vi "[Alternate Method] Extract Data from N-Channel Array (1D Waveform).vi"() -> ()   [LabVIEW 2019]
uses:
  <vilib>/DAQmx/read.llb/DAQmx Read (Analog 1D Wfm NChan NSamp).vi
  <vilib>/DAQmx/create/channels.llb/DAQmx Create Channel (AI-Voltage-Basic).vi
  <vilib>/DAQmx/configure/timing.llb/DAQmx Timing (Sample Clock).vi
  <vilib>/DAQmx/miscellaneous.llb/DAQmx Fill In Error Info.vi
  <resource>/objmgr/daqmx.rc
panel:
  out "Actual Sample Rate (Hz)":dbl
  in  "Desired Sample Rate (Hz)":dbl=2560.0
  in  "Number of Samples":i32=256
  in  "Stop":bool
  out "All Channels":waveform(dbl)[](graph)
  out "Indexed Channel":waveform(dbl)(graph)
  out "Subset of Channels":waveform(dbl)[](graph)
  in  "Physical Channels":tag="PCI-6221/ai0, PCI-6221/ai2:3"
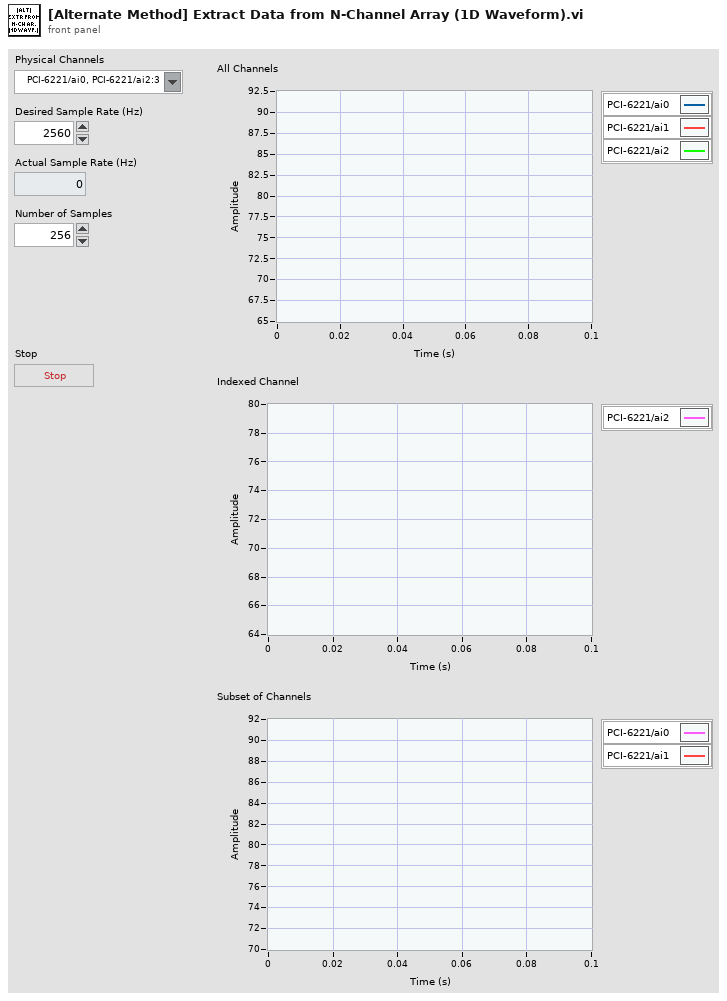
[diagram p1: front panel]
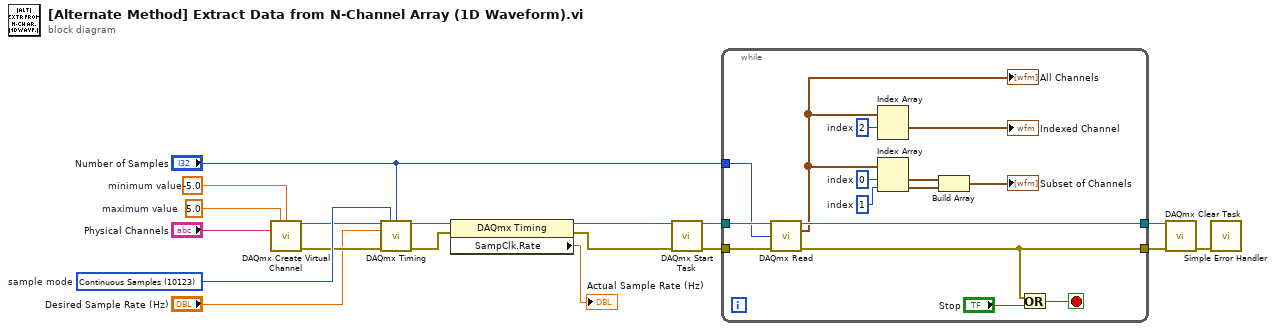
[diagram p0: block diagram]
diagram:
  w13 = 5.0  # maximum value
  w14 = -5.0  # minimum value
  w18 = 10123 items=["Finite Samples"=10178, "Continuous Samples"=10123, "Hardware Timed Single Point"=12522]  # sample mode
  n1 = call-poly <vilib>:"DAQmx Create Virtual Channel.vi"("maximum value"=w13, "minimum value"=w14, "physical channels"="Physical Channels") -> ("task out"=w17:refnum<k21>, "error out"=w16:errorcluster)  [unwired: 11 in]
  n2 = call-poly <vilib>:"DAQmx Timing.vi"("task/channels in"=w17, "sample mode"=w18, "samples per channel"="Number of Samples", "rate"="Desired Sample Rate (Hz)", "error in"=w16) -> ("task out"=w5:refnum<k21>, "error out"=w4:errorcluster)  [unwired: 9 in]
  n3 = property class="DAQmx Timing"(reference=w5, error in=w4) -> (reference out=w3:refnum<k21>, error out=w2:errorcluster, "SampClk.Rate"=→"Actual Sample Rate (Hz)":dbl)
  n4 = call <vilib>:"DAQmx Start Task.vi"("task/channels in"=w3, "error in"=w2) -> ("task out"=w9:refnum<k21>, "error out"=w8:errorcluster)  [unwired: 12 in]
  n5 = while {
    tunnel: [w33] -> w12
    tunnel: [w32] -> w11
    tunnel: w9 -> [w29]
    tunnel: w8 -> [w28]
    tunnel: "Number of Samples" -> [w27]
    stop <- w30 stop-if-true
    w22 = 1  # index
    w23 = 0  # index
    w25 = 2  # index
    n6 = call-poly <vilib>:"DAQmx Read.vi"("task/channels in"=w29, "number of samples per channel"=w27, "error in"=w28) -> ("task out"=w33:refnum<k21>, "data"=w24:waveform(dbl)[], "error out"=w32:errorcluster)  [unwired: 10 in]
    "All Channels" <- w24
    n7 = Index Array "Index Array"(array=w24, index #1=w25) -> (element #1=→"Indexed Channel":waveform(dbl))  [unwired: 1 in, 1 out]
    n8 = Index Array "Index Array"(array=w24, index #1=w23, index #2=w22) -> (element #1=w21:waveform(dbl), element #2=w20:waveform(dbl))
    n9 = Build Array "Build Array"(w21, w20) -> (→"Subset of Channels":waveform(dbl)[])
    n10 = Or(x=w32, y="Stop") -> (x .or. y?=w30:bool)
  }
  n11 = call <vilib>:"DAQmx Clear Task.vi"("task in"=w12, "error in"=w11) -> ("error out"=w10:errorcluster)  [unwired: 13 in]
  n12 = call <vilib>:"Simple Error Handler.vi"("error in (no error)"=w10) -> ()  [unwired: 4 in, 5 out]
